vi "_Remote Communicate.vi"(4 "String":string, 6 "error in (no error)":errorcluster, 7 "DC Param":u16, 9 "Command":T1=enum."Get Info") -> (0 "error out":errorcluster, 1 "Data Array":i32[](array[numeric]), 2 "Info":string, 3 "CommErr":bool)   [LabVIEW 2015]
uses:
  Types/_RT Command.ctl
  Types/TCP Packet Info.ctl
  Global Parameters.vi
  Type/_RT Data.ctl
panel:
  out "Boolean":bool
  in  "Data":T2
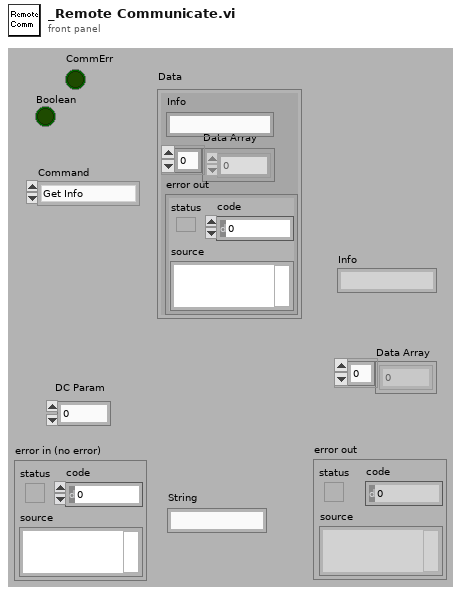
[diagram p1: front panel]
types:
  T1 = typedef "_RT Command.ctl" = enum16{"Start", "Stop", "Get Data", "Get Info", "Get Status"}
  T2 = typedef "_RT Data.ctl" = cluster{"Info":string, "Data Array":i32[], "error out":errorcluster}
  T3 = typedef "TCP Packet Info.ctl" = cluster{"Packet Signature":string, "Sequence Number":i32, "Command":T1, "Data Message Size":u32, "Data Message Size":string, "Data Message":string, "Error Message Size":u32, "Error Message Size":string, "Error Message":string, "Checksum":u32, "Error Message":errorcluster, "Command ID":string}
  T4 = typedef "TCP Packet Info.ctl" = cluster{"Packet Signature":string, "Sequence Number":i32, "Command":T5, "Data Message Size":u32, "Data Message Size":string, "Data Message":string, "Error Message Size":u32, "Error Message Size":string, "Error Message":string, "Checksum":u32, "Error Message":errorcluster, "Command ID":string}
  T5 = typedef "_RT Command.ctl" = enum16{"xml Start Run", "xml Start Actual Run", "xml Stop Run", "xml Runtime Update", "xml Get Status", "xml Get Table", "xml Set Table", "xml Get Configuration", "xml System Status", "xml Set LC Input Logic", "xml Get Data", "xml Get Info", "Start", "StartActualRun", "Stop", "Runtime Update", "Get Data", "Get Info", "Get Status", "Get Param", "Get Config", "Get Table", "Read ADC", "Set Oscillator", "Update Config", "Update Table", "Set All Pol", "Set Pol and DC", "Set Max Mass", "Toggle RP", "Toggle EL", "Set PIC", "Initialize Turbo", "Send Turbo Comm", "Close Turbo", "P1", "P2", "P3", "Send Serial", "Set LC Out", "Get LC In", "Read VAC", "Test Table", "Toggle Power", "Get Startup", "Set Startup", "Get ADC Table", "Set ADC Table", "Get Brief Status", "Get Detail Status", "Auxiliary Update", "Set CC Logics", "Set CC Input Logics", "Ignore Error", "invalid"}
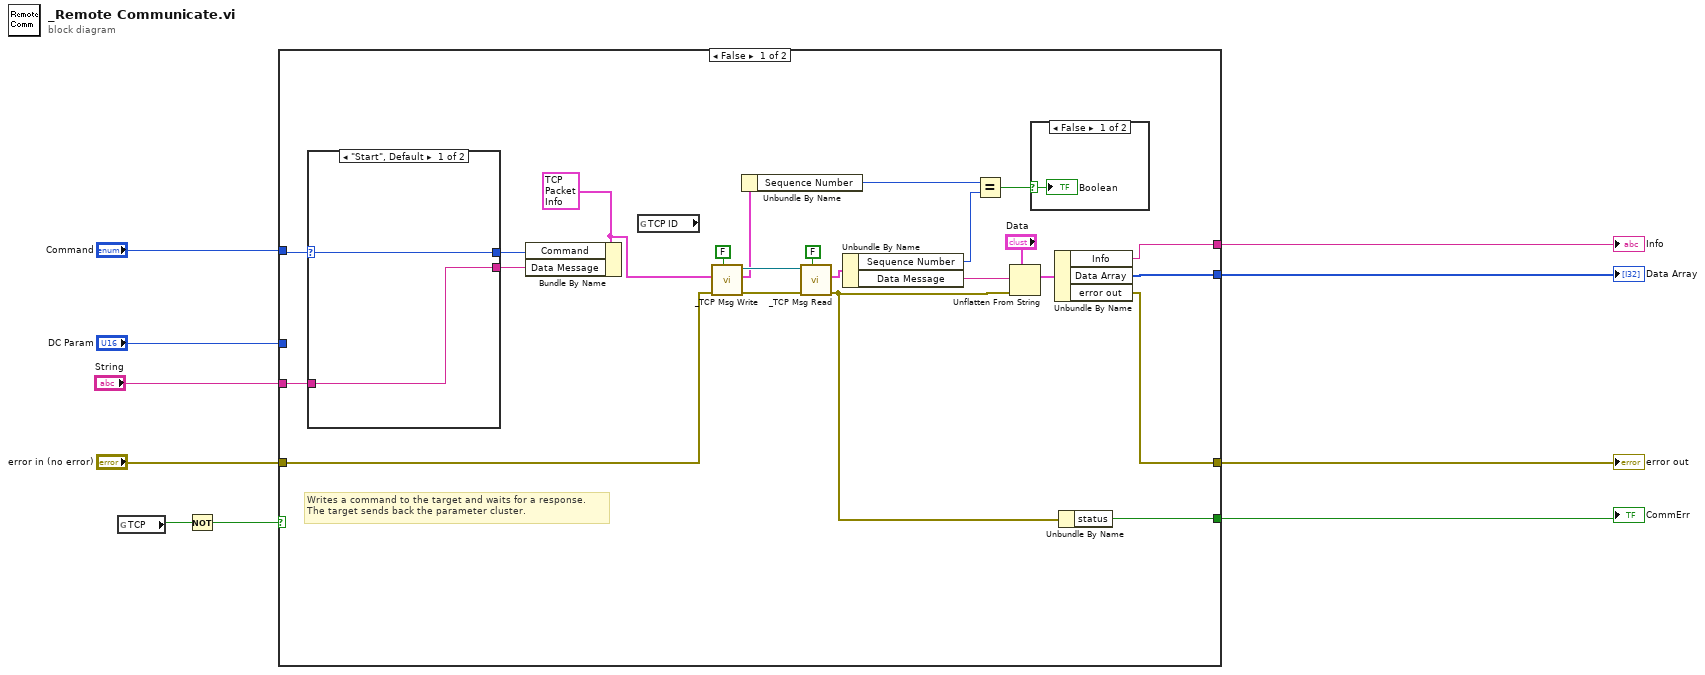
[diagram p0: block diagram]
diagram:
  n1 = global read "Global Parameters.vi" "TCP"() -> (w1:bool)
  n2 = Not(x=w1) -> (.not. x?=w8:bool)
  n3 = case shown="False" w8 {
    selector: w8 -> [_ w38]
    tunnel: [w28 w39] -> w7
    tunnel: "error in (no error)" -> [w25 w39]
    tunnel: [w30 _] -> w5
    tunnel: [w29 _] -> w9
    tunnel: "Command" -> [w15 _]
    tunnel: "DC Param" -> [_ _]
    tunnel: [w27 w38] -> w3
    tunnel: "String" -> [w12 _]
    frame False {
      w11 = T3 {"Packet Signature"="", "Sequence Number"=0, "Command"=enum."Start", "Data Message Size"=0, "Data Message Size"="", "Data Message"="", "Error Message Size"=0, "Error Message Size"="", "Error Message"="", "Checksum"=0, "Error Message"={"status"=FALSE, "code"=0, "source"=""}, "Command ID"=""} ("Packet Info In")
      # "Writes a command to the target and waits for a response.\nThe target sends back the parameter cluster."
      n4 = case shown="\"Start\", Default" w15 {
        selector: w15 -> [w35 w36]
        tunnel: [w35 w36] -> w14
        tunnel: [w34 _] -> w13
        tunnel: w12 -> [w34 _]
        frame "Start", Default {
        }
        frame "Stop" {
        }
      }
      n5 = Bundle By Name(cluster=w11, "Command"=w14, "Data Message"=w13) -> ()  [unwired: 1 out]
      n6 = global read "Global Parameters.vi" "TCP ID"() -> ()  [unwired: 1 out]
      n7 = call "_TCP Msg Write.vi"("RT"=FALSE, "error in"=w25, "Packet Info In"=w11) -> ("error out"=w18:errorcluster, "Packet Info In Out"=w19:T3, "connection ID out"=w32:refnum<k5>)  [unwired: 2 in, 4 out]
      n8 = Unbundle By Name(w19) -> ("Sequence Number"=w22:i32)
      n9 = call "_TCP Msg Read.vi"("RT"=FALSE, "error in"=w18, "connection ID"=w32) -> ("error out"=w16:errorcluster, "Packet Info"=w17:T4)  [unwired: 2 in, 5 out]
      n10 = Unbundle By Name(w17) -> ("Sequence Number"=w21:i32, "Data Message"=w26:string)
      n11 = Equal?(x=w22, y=w21) -> (x = y?=w20:bool)
      n12 = Unflatten From String(type="Data", binary string=w26, error in (no error)=w16) -> (value=w31:T2)  [unwired: 4 out]
      n13 = case shown="False" w20 {
        selector: w20 -> [w37 _]
        frame False {
          "Boolean" <- w37
        }
        frame True {
        }
      }
      n14 = Unbundle By Name(w31) -> ("Info"=w30:string, "Data Array"=w29:i32[], "error out"=w28:errorcluster)
      n15 = Unbundle By Name(w16) -> ("status"=w27:bool)
    }
    frame True {
    }
  }
  "error out" <- w7
  "Data Array" <- w9
  "Info" <- w5
  "CommErr" <- w3
